vi "MainCode.vi"() -> ()   [LabVIEW 2020]
uses:
  Subs/SystemLink/SL_Subs/SL_XControl.xctl
  Subs/ColorText/Code.xctl
  Subs/SystemLink/SL_Subs/SystemLink_Write_String.vi
panel:
  in  "Code":string(xcontrol)
  in  "Path to keras folder":path
  out "Labels":string="0 go\n1 stop\n2 right\n3 nothing\n"
  in  "SystemLink":string(xcontrol)="fred"
  out "Percentages":u8[](array[slide])=[0, 99, 1, 0] scale=0.0..100.0
  in  "Camera Params":T1={"plane"="RGB", "zoom"=0.520408163265306, "rotation"=0} {"rotation" scale=0.0..180.0; "zoom" scale=0.0..1.0}
  out "picture":picture
  out "dt":u32=141
  in  "stop":bool
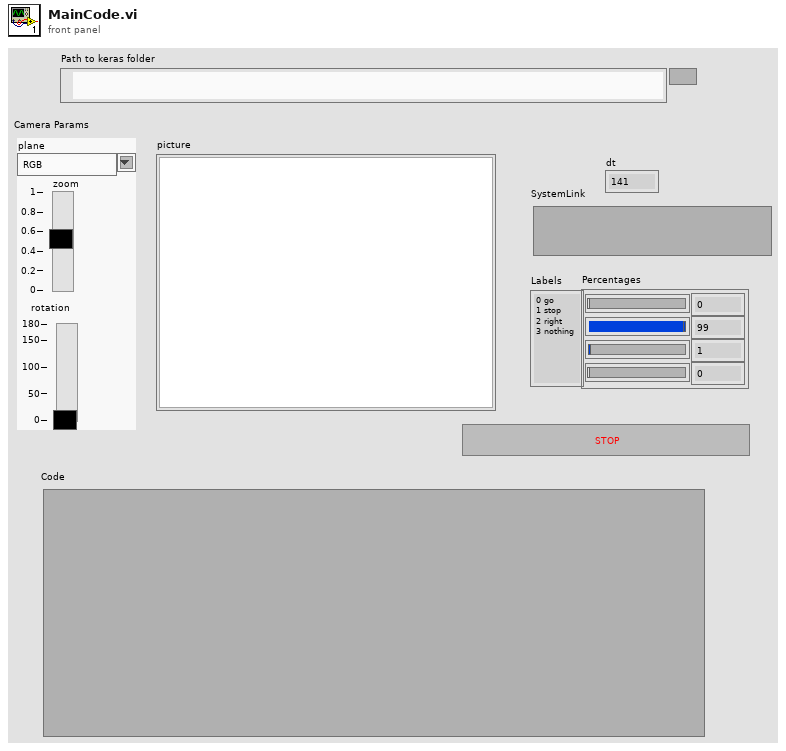
[diagram p1: front panel]
types:
  T1 = cluster{"plane":string, "zoom":dbl, "rotation":u8}
  T2 = cluster{"session":refnum<k35>, "OpenCV":path, "Tensor Flow":path, "Image":path, "Labels":string}
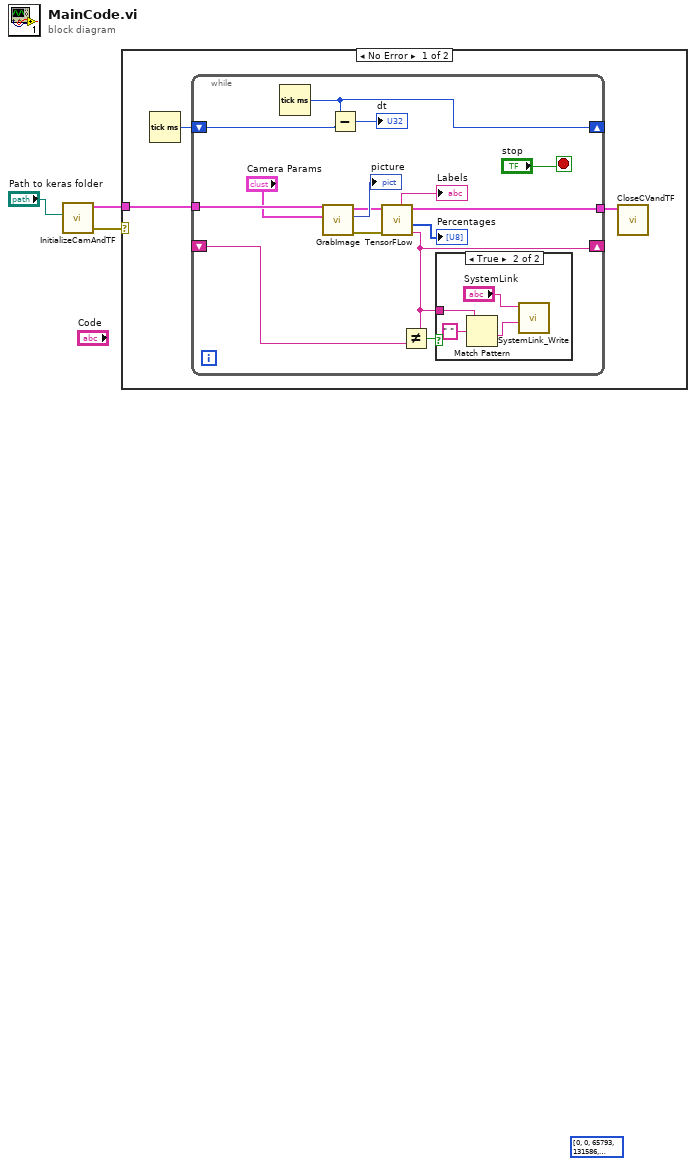
[diagram p0: block diagram]
diagram:
  (unwired) u32[] [0, 0, 65793, 131586, 197379, 263171, 328965, 394758, 460551, 526344, 592137, 657930, 723723, 789516, 855309, 921102, 986895, 1052688, 1118481, 1184274, 1250067, 1315860, 1381653, 1447446, 1513239, 1579032, 1644825, 1710618, 1776411, 1842204, 1907997, 1973790, 2039583, 2105376, 2171169, 2236962, 2302755, 2368548, 2434341, 2500134, 2565927, 2631720, 2697513, 2763306, 2829099, 2894892, 2960685, 3026478, 3092271, 3158064, 3223857, 3289650, 3355443, 3421236, 3487029, 3552822, 3618615, 3684408, 3750201, 3815994, 3881787, 3947580, 4013373, 4079166, 4144959, 4210752, 4276545, 4342338, 4408131, 4473924, 4539717, 4605510, 4671303, 4737096, 4802889, 4868682, 4934475, 5000268, 5066061, 5131854, 5197647, 5263440, 5329233, 5395026, 5460819, 5526612, 5592405, 5723991, 5789784, 5855577, 5921370, 5987163, 6052956, 6118749, 6184542, 6250335, 6316128, 6381921, 6447714, 6513507, 6579300, 6645093, 6710886, 6776679, 6842472, 6908265, 6974058, 7039851, 7105644, 7171437, 7237230, 7303023, 7368816, 7434609, 7500402, 7566195, 7631988, 7697781, 7763574, 7829367, 7895160, 7960953, 8026746, 8092539, 8158332, 8224125, 8289918, 8355711, 8421504, 8487297, 8553090, 8618883, 8684676, 8750469, 8816262, 8882055, 8947848, 9013641, 9079434, 9145227, 9211020, 9276813, 9342606, 9408399, 9474192, 9539985, 9605778, 9671571, 9737364, 9803157, 9868950, 9934743, 10000536, 10066329, 10132122, 10197915, 10263708, 10329501, 10395294, 10461087, 10526880, 10592673, 10658466, 10724259, 10790052, 10855845, 10921638, 10987431, 11053224, 11119017, 11184810, 11250603, 11382189, 11447982, 11513775, 11579568, 11645361, 11711154, 11776947, 11842740, 11908533, 11974326, 12040119, 12105912, 12171705, 12237498, 12303291, 12369084, 12434877, 12500670, 12566463, 12632256, 12698049, 12763842, 12829635, 12895428, 12961221, 13027014, 13092807, 13158600, 13224393, 13290186, 13355979, 13421772, 13487565, 13553358, 13619151, 13684944, 13750737, 13816530, 13882323, 13948116, 14013909, 14079702, 14145495, 14211288, 14277081, 14342874, 14408667, 14474460, 14540253, 14606046, 14671839, 14737632, 14803425, 14869218, 14935011, 15000804, 15066597, 15132390, 15198183, 15263976, 15329769, 15395562, 15461355, 15527148, 15592941, 15658734, 15724527, 15790320, 15856113, 15921906, 15987699, 16053492, 16119285, 16185078, 16250871, 16316664, 16382457, 16448250, 16514043, 16579836, 16645629, 16711422, 16777215, 16777215] ("Greyscale")
  n1 = call "InitializeCamAndTF.vi"("Path to keras folder"="Path to keras folder") -> ("error out"=w2:errorcluster, "TFinfo out"=w3:T2)  [unwired: 9 in]
  n2 = case shown="No Error" w2 {
    tunnel: w3 -> [w6 _]
    frame No Error {
      n3 = Tick Count (ms)() -> (millisecond timer value=w5:u32)
      n4 = while {
        tunnel: w6 -> [w15]
        shift-right: [w21] -> _
        shift-left: w5 -> [w20]
        tunnel: [w12] -> w4
        shift-right: [w8] -> _
        shift-left: _ -> [w7]
        stop <- "stop" stop-if-true
        n5 = Tick Count (ms)() -> (millisecond timer value=w21:u32)
        n6 = call "GrabImage.vi"("Camera Params"="Camera Params", "TFinfo In"=w15) -> ("error out"=w17:errorcluster, "new picture"=→"picture":picture, "TFinfo out"=w13:T2)  [unwired: 7 in]
        n7 = Subtract(x=w21, y=w20) -> (x-y=→"dt":u32)
        n8 = call "TensorFLow.vi"("error in (no error)"=w17, "TFinfo In"=w13) -> ("Label"=w8:string, "Percentages"=→"Percentages":u8[], "TFinfo out"=w12:T2, "Labels"=→"Labels":string)  [unwired: 5 in, 1 out]
        n9 = Not Equal?(x=w8, y=w7) -> (x != y?=w9:bool)
        n10 = case shown="True" w9 {
          tunnel: w8 -> [_ w24]
          frame False {
          }
          frame True {
            n11 = Match Pattern(string=w24, regular expression=" ") -> (after substring=w23:string)  [unwired: 1 in, 3 out]
            n12 = call-poly "SystemLink_Write.vi"("String"=w23, "SL_XControl"="SystemLink") -> ()  [unwired: 10 in]
          }
        }
      }
      n13 = call "CloseCVandTF.vi"("TFinfo In"=w4) -> ()  [unwired: 10 in, 1 out]
    }
    frame Error {
    }
  }
